vi "Get All Nodes.vi"(8 "error in (no error)":errorcluster, 11 "map reference in":refnum<data-value>) -> (0 "error out":errorcluster, 2 "nodes":cluster{"name":string, "coordinates":dbl[]}[](array[cluster]), 3 "map reference out":refnum<data-value>)   [LabVIEW 2017, in "NI_Robotics_DirectedGraphWorldMap.lvclass"]
doc: "Returns the names and coordinates of all <B>nodes</B> defined in a map."
uses:
  <vilib>/robotics/Navigation/shared/WorldMap/DirectedGraphWorldMap/NI_Robotics_DirectedGraphWorldMap.lvclass
  <vilib>/robotics/Navigation/shared/WorldMap/DirectedGraphWorldMap/NI_Robotics_DirectedGraphWorldMap.lvclass/NI_Robotics_DirectedGraphWorldMap.ctl
  <vilib>/robotics/Navigation/shared/MapNode/DirectedGraphMapNode/NI_Robotics_DirectedGraphMapNode.lvclass
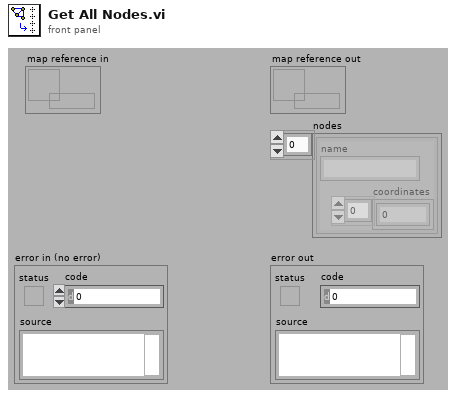
[diagram p1: front panel]
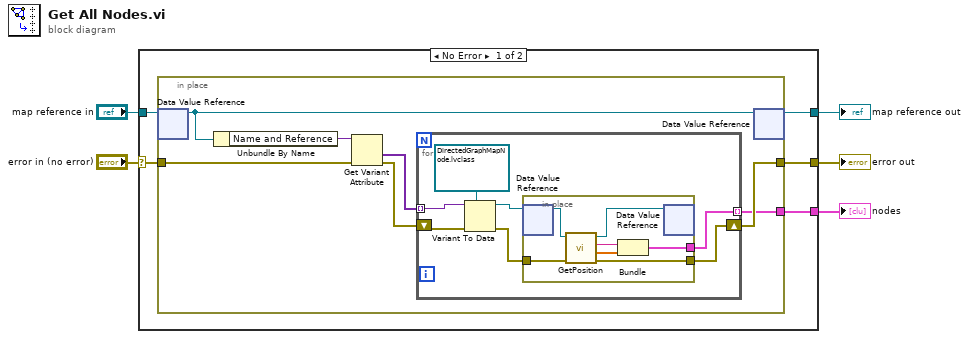
[diagram p0: block diagram]
diagram:
  n1 = case shown="No Error" "error in (no error)" {
    selector: "error in (no error)" -> [w9 w33]
    tunnel: [w8 w33] -> w4
    tunnel: "map reference in" -> [w10 w32]
    tunnel: [w7 _] -> w2
    tunnel: [w6 w32] -> w1
    frame No Error {
      n2 = in-place {
        in-place-border: w9 -> [w15]
        in-place-border: [w13] -> w8
        in-place-border: [w11] -> w7
        n3 = in-place-dvr #1(w10) -> (w17:refnum<class "NI_Robotics_DirectedGraphWorldMap.lvclass">)  [unwired: 1 out]
        n4 = Unbundle By Name(w17) -> ("Name and Reference"=w16:variant)
        n5 = Get Variant Attribute(Variant=w16, error in=w15) -> (values=w12:variant[], error out=w14:errorcluster)  [unwired: 2 in, 2 out]
        n6 = for {
          tunnel: w12 -> [w23] mode=indexing
          shift-right: [w20] -> w13
          shift-left: w14 -> [w24]
          tunnel: [w18] -> w11 mode=indexing
          n7 = Variant To Data(error in=w24, type=refnum<data-value> refnum ("Node ref"), Variant=w23) -> (data=w19:refnum<data-value>, error out=w21:errorcluster)
          n8 = in-place {
            in-place-border: w21 -> [w31]
            in-place-border: [w30] -> w20
            in-place-border: [w25] -> w18
            n9 = in-place-dvr #2(w19) -> (w29:refnum<class "NI_Robotics_DirectedGraphMapNode.lvclass">)  [unwired: 1 out]
            n10 = call <vilib>:"GetPosition.vi"("error in (no error)"=w31, "DirectedGraphMapNode in"=w29) -> ("error out"=w30:errorcluster, "coordinates"=w26:dbl[], "name"=w27:string, "DirectedGraphMapNode out"=w28:refnum<class "NI_Robotics_DirectedGraphMapNode.lvclass">)  [unwired: 6 in]
            n11 = Bundle("name"=w27, "coordinates"=w26) -> (w25:cluster{"name":string, "coordinates":dbl[]})  [unwired: 1 in]
            n12 = in-place-dvr #2(w28) -> ()  [unwired: 2 out]
          }
        }
        n13 = in-place-dvr #1(w17) -> (w6:refnum<data-value>)  [unwired: 1 out]
      }
    }
    frame Error {
    }
  }
  "error out" <- w4
  "nodes" <- w2
  "map reference out" <- w1
